vi "GetFunction_XDM3051.vi"(8 "error in":errorcluster, 11 "RS232_Input":refnum<visa-resource-name>) -> (0 "error out":errorcluster, 2 "response":string, 3 "RS232_Output":refnum<visa-resource-name>)   [LabVIEW 2017]
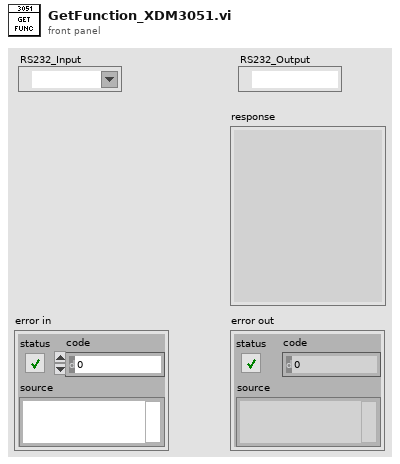
[diagram p1: front panel]
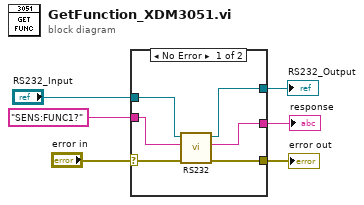
[diagram p0: block diagram]
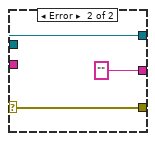
[diagram p2: hidden frame]
diagram:
  n1 = case shown="No Error" "error in" {
    selector: "error in" -> [w7 w15]
    tunnel: [w12 w15] -> w5
    tunnel: "RS232_Input" -> [w11 w14]
    tunnel: "SENS:FUNC1?" ("command") -> [w8 _]
    tunnel: [w10 "" ("response")] -> w2
    tunnel: [w9 w14] -> w1
    frame No Error {
      n2 = call "RS232.vi"("error in"=w7, "command"=w8, "RS232_Input"=w11) -> ("error out"=w12:errorcluster, "response"=w10:string, "RS232_Output"=w9:refnum<visa-resource-name>)  [unwired: 6 in]
    }
    frame Error {
    }
  }
  "error out" <- w5
  "RS232_Output" <- w1
  "response" <- w2
